vi "Elettrotest60A Read.vi"(5 "Dato-1":dbl, 7 "error in":errorcluster, 8 "String command":string, 10 "VISA resource name in":refnum<visa-resource-name>) -> (0 "error out":errorcluster, 1 "Converted":dbl, 2 "Stop":bool, 3 "VISA resource name out":refnum<visa-resource-name>, 4 "FS 2":T1={"Resistenza1"=2.0, "Resistenza2"=2.0, "RESISTENZA"=2.0})   [LabVIEW 2019]
panel:
  out "return count":u32
  in  "FS":T1={"Resistenza1"=2.0, "Resistenza2"=2.0, "RESISTENZA"=2.0}
  out "String command 2":string
  # "Deve essere compreso\ntra 1 e 9"
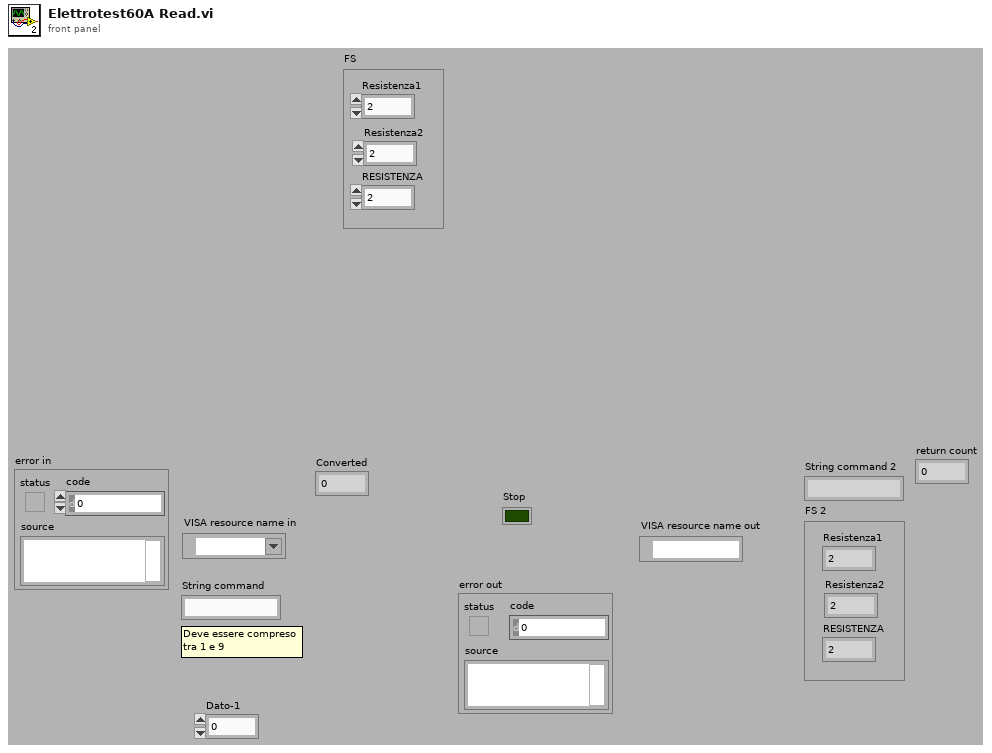
[diagram p1: front panel]
types:
  T1 = cluster{"Resistenza1":dbl, "Resistenza2":dbl, "RESISTENZA":dbl}
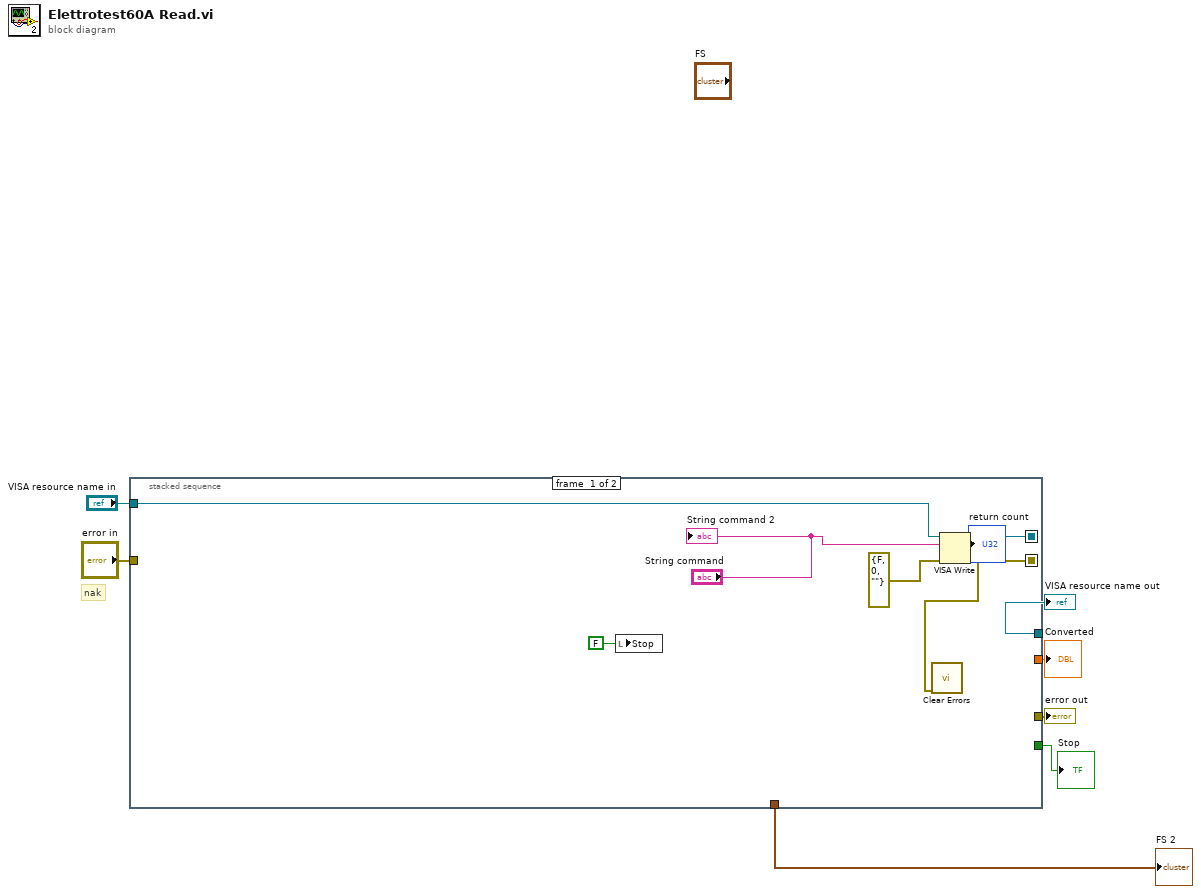
[diagram p0: block diagram]
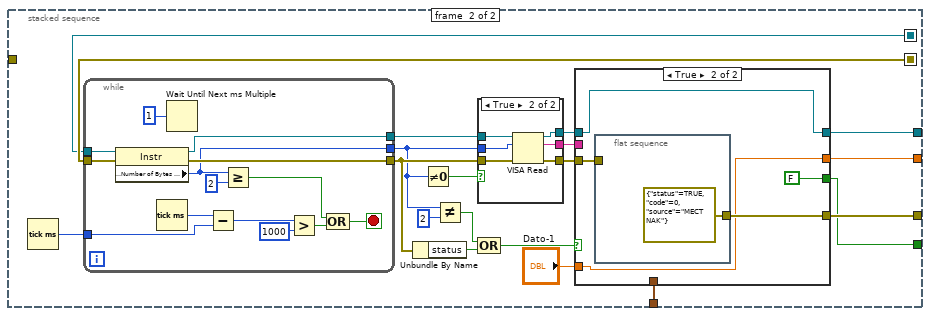
[diagram p2: hidden frame]
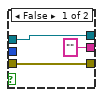
[diagram p3: hidden frame]
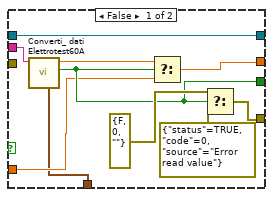
[diagram p4: hidden frame]
diagram:
  # "nak"
  n1 = stacked-sequence {
    seq-local: [w14 _] -> [_ w27]
    seq-local: [w9 _] -> [_ w34]
    tunnel: [_ w29] -> w6
    tunnel: "VISA resource name in" -> [w13 _]
    tunnel: [_ w33] -> w5
    tunnel: "error in" -> [_ _]
    tunnel: [_ w28] -> w3
    tunnel: [_ w18] -> w2
    tunnel: [_ w15] -> w1
    frame #0 {
      n2 = local write "Stop"(FALSE ("Stop")) -> ()
      n3 = VISA Write(VISA resource name=w13, write buffer="String command", error in (no error)=errorcluster {"status"=FALSE, "code"=0, "source"=""}) -> (VISA resource name out=w14:refnum<visa-resource-name>, return count=→"return count":u32, error out=w9:errorcluster)
      n4 = call <vilib>:"Clear Errors.vi"("error in (no error)"=w9) -> ()  [unwired: 5 in, 2 out]
      "String command 2" <- "String command"
    }
    frame #1 {
      n5 = Tick Count (ms)() -> (millisecond timer value=w30:u32)
      n6 = while {
        tunnel: w27 -> [w57]
        tunnel: w34 -> [w56]
        tunnel: [w52] -> w24
        tunnel: [w48] -> w20
        tunnel: [w51] -> w25
        tunnel: w30 -> [w45]
        stop <- w46 stop-if-true
        n7 = property class="Instr"(reference=w57, error in=w56) -> (reference out=w51:refnum<visa-resource-name>, error out=w52:errorcluster, "Serial Settings:Number of Bytes at Serial Port"=w48:u32)
        n8 = Tick Count (ms)() -> (millisecond timer value=w55:u32)
        n9 = Wait Until Next ms Multiple(millisecond multiple=u32 1) -> ()  [unwired: 1 out]
        n10 = Subtract(x=w55, y=w45) -> (x-y=w54:u32)
        n11 = Greater Or Equal?(x=w48, y=2) -> (x >= y?=w47:bool)
        n12 = Greater?(x=w54, y=1000) -> (0:w50:bool)
        n13 = Compound Arithmetic op=OR(w47, w50) -> (w46:bool)
      }
      n14 = Unbundle By Name(w24) -> ("status"=w26:bool)
      n15 = Not Equal To 0?(x=w20) -> (x != 0?=w21:bool)
      n16 = Not Equal?(x=w20, y=2) -> (x != y?=w31:bool)
      n17 = case shown="True" w21 {
        tunnel: w25 -> [w37 w43]
        tunnel: w24 -> [w36 w42]
        tunnel: [w37 w41] -> w23
        tunnel: [w36 w40] -> w22
        tunnel: w20 -> [_ w39]
        tunnel: ["" ("read buffer") w38] -> w19
        frame False {
        }
        frame True {
          n18 = VISA Read(VISA resource name=w43, byte count=w39, error in (no error)=w42) -> (VISA resource name out=w41:refnum<visa-resource-name>, read buffer=w38:string, error out=w40:errorcluster)  [unwired: 1 out]
        }
      }
      n19 = Compound Arithmetic op=OR(w31, w26) -> (w17:bool)
      n20 = case shown="True" w17 {
        tunnel: [w62 w72] -> w29
        tunnel: [w67 w71] -> w33
        tunnel: w23 -> [w67 w71]
        tunnel: w22 -> [_ w70]
        tunnel: [w65 w68] -> w28
        tunnel: w19 -> [w66 _]
        tunnel: [w60 FALSE ("Check last 2bit(T=OK)")] -> w18
        tunnel: "Dato-1" -> [w59 w68]
        tunnel: [w58 _] -> w15
        frame False {
          n21 = call "Converti_ dati Elettrotest60A.vi"("String in"=w66) -> ("Check last 2bit(T=OK)"=w60:bool, "Converted"=w64:dbl, "FS 2"=w58:T1)  [unwired: 8 out]
          n22 = Select(t=w64, s=w60, f=w59) -> (s? t:f=w65:dbl)
          n23 = Select(t=errorcluster {"status"=FALSE, "code"=0, "source"=""} ("error out 2"), s=w60, f=errorcluster {"status"=TRUE, "code"=0, "source"="Error read value"} ("error out 2")) -> (s? t:f=w62:errorcluster)
        }
        frame True {
          n24 = flat-sequence {
            tunnel: [errorcluster {"status"=TRUE, "code"=0, "source"="MECT NAK"} ("error out 2")] -> w72
            tunnel: w70 -> [_]
            frame #0 {
            }
          }
        }
      }
    }
  }
  "error out" <- w6
  "VISA resource name out" <- w5
  "Converted" <- w3
  "Stop" <- w2
  "FS 2" <- w1
